vi "Mask Write Register.vi"(4 "OR Mask":u16, 6 "AND Mask":u16, 8 "error in":errorcluster, 10 "address":u16, 11 "Master CR in":refnum<class "WebSocket Client CR.lvclass">) -> (0 "error out":errorcluster, 3 "Master CR out":refnum<class "WebSocket Client CR.lvclass">)   [LabVIEW 2021]
doc: "Writes the masked value of a single register using an <b>AND mask</b> and an <b>OR mask</b> using the equation below:\nResult=(Current Value AND AndMask) OR (OrMask AND !AndMask)"
uses:
  WebSocket Client CR.lvclass
  WebSocket Client CR.lvclass/WebSocket Client CR.ctl
  Modbus_v121c/Data Model/Device Data Model.lvclass
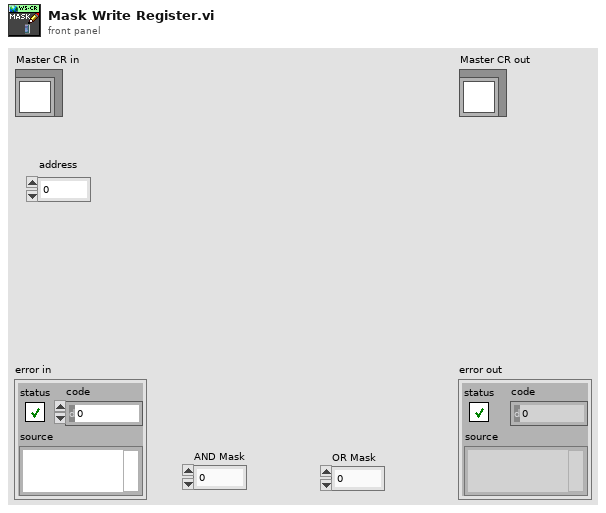
[diagram p1: front panel]
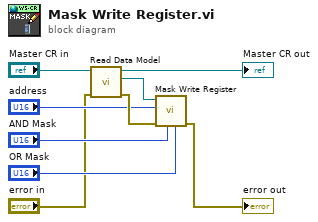
[diagram p0: block diagram]
diagram:
  n1 = call "Read Data Model.vi"("error in (no error)"="error in", "Master CR in"="Master CR in") -> ("error out"=w6:errorcluster, "Data Model"=w7:refnum<class "Device Data Model.lvclass">, "Master CR out"=→"Master CR out":refnum<class "WebSocket Client CR.lvclass">)  [unwired: 7 in]
  n2 = call-dynamic "Mask Write Register.vi"("OR Mask"="OR Mask", "AND Mask"="AND Mask", "error in"=w6, "address"="address", "device data model in"=w7) -> ("error out"=→"error out":errorcluster)  [unwired: 5 in, 1 out]
